vi "Write Transient Stimulus Parameter.vi"(8 "error in (no error)":errorcluster, 10 "Stimulus Parameters":T1, 11 "Data Analyser Report in":refnum<class "Data Analyser Report.lvclass">) -> (0 "error out":errorcluster, 3 "Data Analyser Report out":refnum<class "Data Analyser Report.lvclass">)   [LabVIEW 2016, in "Data Analyser Report.lvclass"]
uses:
  Data Analyser Report.lvclass
  C:/Users/w.figtree/Desktop/Work/4. Projects/3. In Progress Engineering Projects/EMA/src/core/Classes/Excel Interface/Excel Sheet/Excel Sheet.lvclass
  Excel Interface/Excel Sheet/Write to Cell - Int.vi
  Excel Interface/Excel Sheet/Excel Sheet.lvclass
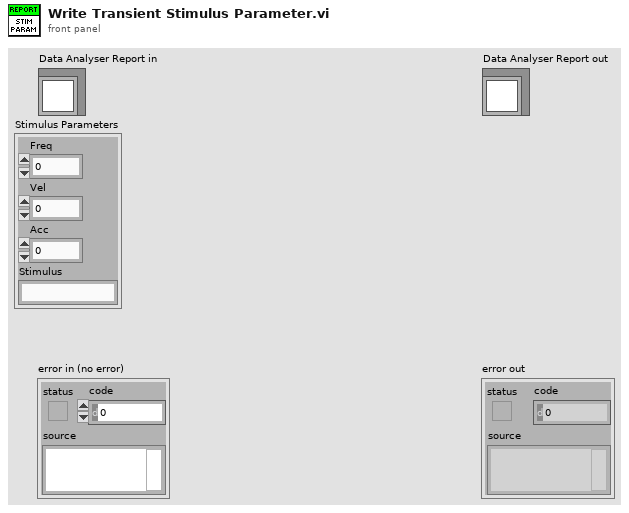
[diagram p1: front panel]
types:
  T1 = cluster{"Freq":dbl, "Vel":i32, "Acc":i32, "Stimulus":string}
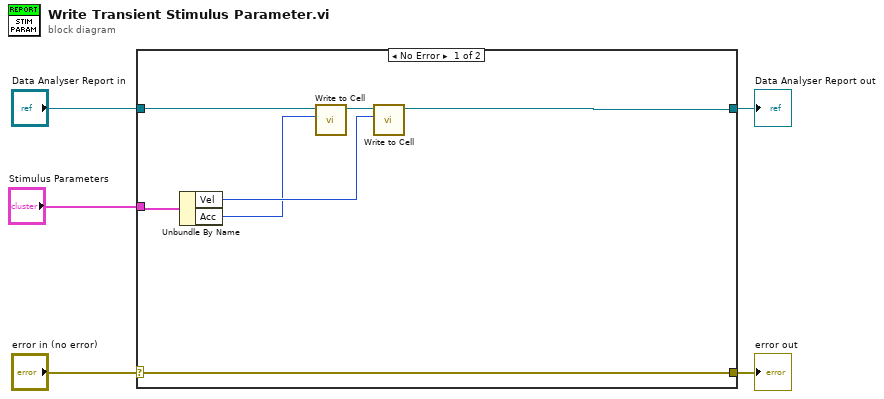
[diagram p0: block diagram]
diagram:
  n1 = case shown="No Error" "error in (no error)" {
    selector: "error in (no error)" -> [w12 w14]
    tunnel: [w12 w14] -> w4
    tunnel: [w7 w13] -> w2
    tunnel: "Data Analyser Report in" -> [w10 w13]
    tunnel: "Stimulus Parameters" -> [w11 _]
    frame No Error {
      n2 = Unbundle By Name(w11) -> ("Vel"=w9:i32, "Acc"=w8:i32)
      n3 = call-poly "Write to Cell.vi"("Value"=w8, "Excel Sheet in"=w10) -> ("Excel Sheet out"=w6:refnum<class "Data Analyser Report.lvclass">)  [unwired: 9 in]
      n4 = call-poly "Write to Cell.vi"("Value"=w9, "Excel Sheet in"=w6) -> ("Excel Sheet out"=w7:refnum<class "Data Analyser Report.lvclass">)  [unwired: 9 in]
    }
    frame Error {
    }
  }
  "error out" <- w4
  "Data Analyser Report out" <- w2
